vi "EE_DataAcquisitionLoop.vi"(8 "error in (no error)":errorcluster, 9 "StopButton Ref":refnum<vi>, 10 "RawDataQueue in":T1, 11 "EmotivEpocHeadsetControls in":refnum<class "EmotivEpocHeadsetControls.lvclass">) -> (0 "error out":errorcluster, 2 "RawDataQueue out":T1, 3 "EmotivEpocHeadsetControls out":refnum<class "EmotivEpocHeadsetControls.lvclass">)   [LabVIEW 2016, in "Emotiv Epoc.lvlib" / "EmotivEpocHeadsetControls.lvclass"]
uses:
  EmotivEpocHeadsetControls.lvclass
  EE_Queue_Refnum.ctl
  EE_Queue_Data_Type.ctl
  EE_SignalStrength_enum.ctl
  EE_EEG_ContactQuality_enum.ctl
  EmotivEpocHeadsetControls.lvclass/EmotivEpocHeadsetControls.ctl
  <vilib>/Platform/TimedLoop/XDataNode/timing_clust.ctl
  <vilib>/Platform/TimedLoop/XDataNode/nitl_modes.ctl
  <vilib>/Platform/TimedLoop/XDataNode/wakeup.ctl
  <vilib>/Platform/TimedLoop/XDataNode/XDataNode.xnode
  <vilib>/Platform/TimedLoop/XDataNode/XDNodeRunTimeDep.lvlib
  Emotiv Epoc.lvlib
panel:
  # "This VI is a part of BCI Design library, http://www.ru-bci.org \nCopyright © 2020, Sotnikov Peter, All rights reserved. License: CC BY-NC 4.0"
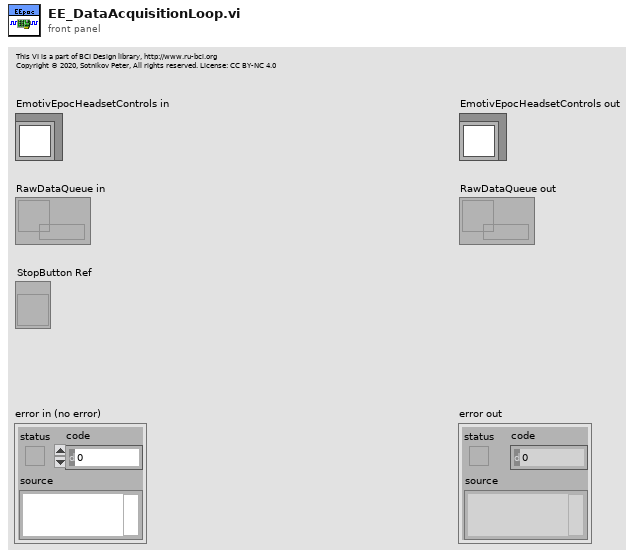
[diagram p1: front panel]
types:
  T1 = typedef "Emotiv Epoc.lvlib/EE_Queue_Refnum.ctl" = refnum<queue>
  T2 = typedef "Emotiv Epoc.lvlib/EE_Queue_Data_Type.ctl" = cluster{"FinishedLate?":bool, "UserActive?":bool, "WirelessSignalStatus":T3, "EDK_ERROR_CODE":i32, "nSampleOut":u32, "CurrentTimestamp":timestamp, "RawChannelsData ":dbl[][], "EEG_ContactsQuality":T4[]}
  T3 = typedef "Emotiv Epoc.lvlib/EmotivEpocHeadsetControls.lvclass/EE_SignalStrength_enum.ctl" = enum32{"NO_SIGNAL", "BAD_SIGNAL", "GOOD_SIGNAL"}
  T4 = typedef "Emotiv Epoc.lvlib/EE_EEG_ContactQuality_enum.ctl" = enum16{"EEG_CQ_NO_SIGNAL", "EEG_CQ_VERY_BAD", "EEG_CQ_POOR", "EEG_CQ_FAIR", "EEG_CQ_GOOD"}
  T5 = typedef "XDNodeRunTimeDep.lvlib/timing_clust.ctl" = cluster{"Expected End [f-1]":u64, "Actual End [f-1]":u64, "Finished Late? [f-1]":bool, "Expected End [i-1]":u64, "Actual End [i-1]":u64, "Finished Late? [i-1]":bool, "Expected Start [i]":u64, "Actual Start [i]":u64, "Expected Start [f]":u64, "Actual Start [f]":u64, "Source Name":string, "Structure Name":string, "Period":i64, "Deadline":i64, "Offset":i64, "Start":i64, "Priority":i32, "Timeout":i32, "Mode":T6, "Wakeup Reason":T7, "Error":errorcluster, "Source Type":string, "Secondary Source Type":string, "Global End Time":u64, "Global Start Time":u64, "Frame Duration":u64, "Iteration Duration":u64, "Assigned CPU":i32, "I/O Scan Engine Mode":u32}
  T6 = typedef "XDNodeRunTimeDep.lvlib/nitl_modes.ctl" = enum32{"No Change", "Process missed periods, maintain original phase", "Discard missed periods, maintain original phase", "Process missed periods, ignore original phase", "Discard missed periods, ignore original phase"}
  T7 = typedef "XDNodeRunTimeDep.lvlib/wakeup.ctl" = enum32{"Normal", "Aborted", "Asynchronous wakeup", "Timing source error", "Timed loop error", "Timeout"}
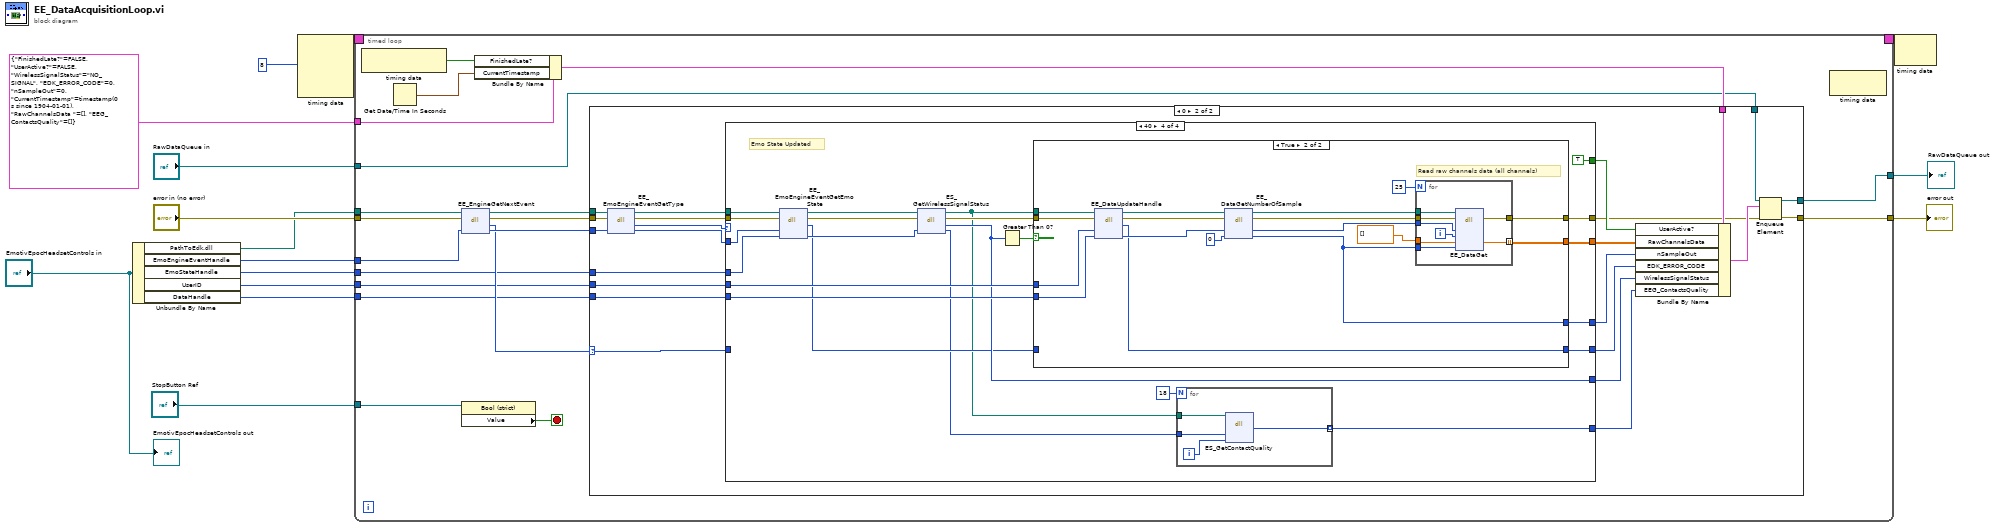
[diagram p0: block diagram]
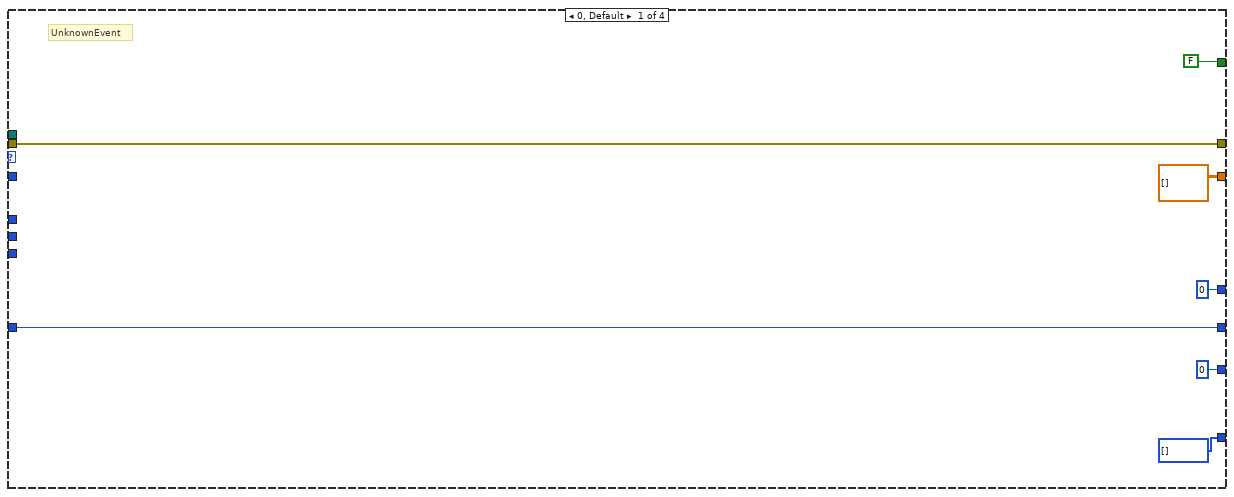
[diagram p3: hidden frame]
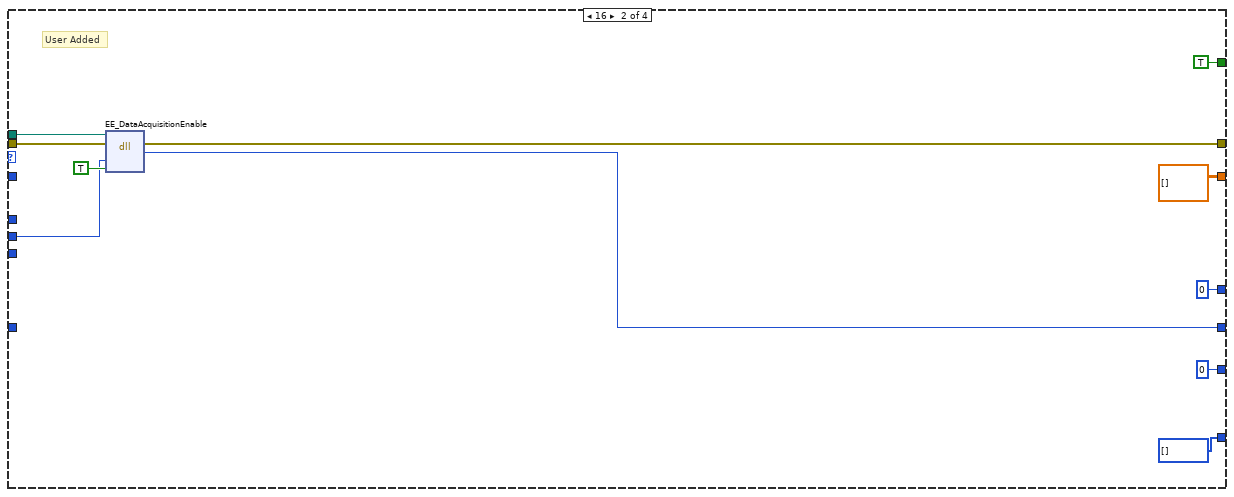
[diagram p4: hidden frame]
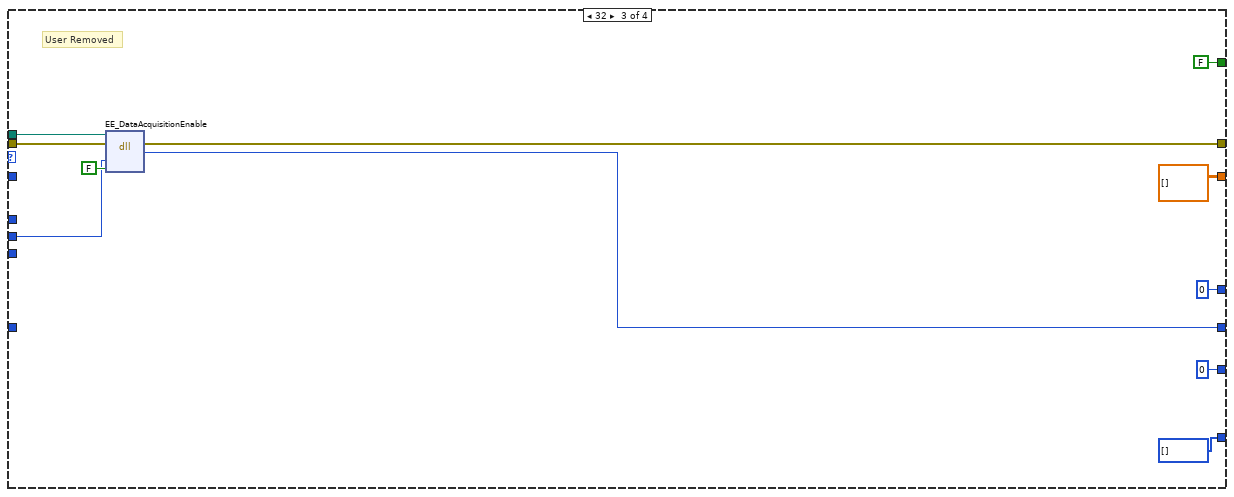
[diagram p5: hidden frame]
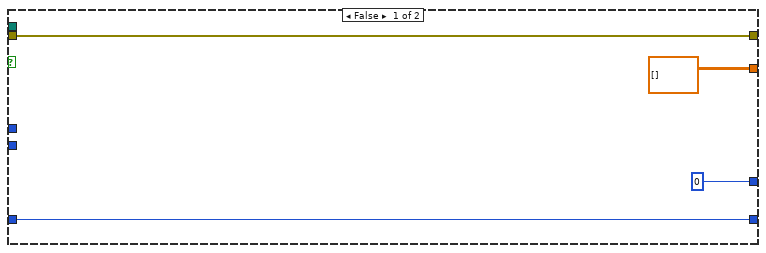
[diagram p6: hidden frame]
diagram:
  n1 = Unbundle By Name("EmotivEpocHeadsetControls in") -> ("PathToEdk.dll"=w10:path, "EmoEngineEventHandle"=w8:i64, "EmoStateHandle"=w5:i64, "UserID"=w6:u32, "DataHandle"=w4:i64)
  n2 = node-c288(i64 8 ("Period")) -> (w15:T5)  [unwired: 3 in]
  n3 = timed-loop {
    timing: w15 -> [_]
    timing-out: [_] -> w14
    tunnel: "error in (no error)" -> [w30]
    tunnel: "RawDataQueue in" -> [w18]
    tunnel: w10 -> [w29]
    tunnel: [w17] -> w9
    tunnel: w8 -> [w27]
    tunnel: "StopButton Ref" -> [w26]
    tunnel: w6 -> [w25]
    tunnel: w5 -> [w24]
    tunnel: w4 -> [w23]
    tunnel: T2 {"FinishedLate?"=FALSE, "UserActive?"=FALSE, "WirelessSignalStatus"=enum."NO_SIGNAL", "EDK_ERROR_CODE"=0, "nSampleOut"=0, "CurrentTimestamp"=timestamp(0 s since 1904-01-01), "RawChannelsData "=[], "EEG_ContactsQuality"=[]} ("Queue_Data_Type") -> [w22]
    tunnel: [w16] -> w1
    stop <- w34 stop-if-true
    n4 = node-c288() -> (w21:bool)  [unwired: 1 in]
    n5 = Get Date/Time In Seconds() -> (seconds since 1Jan1904=w20:timestamp)
    n6 = dll-call lib="?" fn="EE_EngineGetNextEvent"(path in=w29, error in=w30, "EmoEngineEventHandle"=w27) -> (path out=w32:path, error out=w31:errorcluster, "EDK_ERROR_CODE"=w28:i32, "EmoEngineEventHandle"=w33:i64)  [unwired: 1 in]
    n7 = property class="Bool (strict)"(reference=w26) -> ("Value"=w34:bool)  [unwired: 1 in, 2 out]
    n8 = Bundle By Name(cluster=w22, "FinishedLate?"=w21, "CurrentTimestamp"=w20) -> (w19:T2)
    n9 = case shown="0" w28 {
      selector: w28 -> [_ w49]
      tunnel: w33 -> [_ w55]
      tunnel: w32 -> [_ w54]
      tunnel: w31 -> [w36 w53]
      tunnel: [w36 w42] -> w17
      tunnel: w25 -> [_ w52]
      tunnel: w24 -> [_ w51]
      tunnel: w23 -> [_ w50]
      tunnel: w19 -> [_ w47]
      tunnel: w18 -> [w35 w46]
      tunnel: [w35 w45] -> w16
      frame 1536, Default {
        # "There are no new EmoEngine events at this time"
      }
      frame 0 {
        n10 = dll-call lib="C:/Program Files/Emotiv Development Kit_v1.0.0.3-PREMIUM/edk.dll" fn="EE_EmoEngineEventGetType"(path in=w54, error in=w53, "EmoEngineEventHandle"=w55) -> (path out=w58:path, error out=w57:errorcluster, "EE_Event_type"=w56:u32, "EmoEngineEventHandle"=w59:i64)  [unwired: 1 in]
        n11 = case shown="40" w56 {
          tunnel: w57 -> [w66 w77 w88 w110]
          tunnel: w58 -> [_ w76 w87 w109]
          tunnel: [w66 w75 w86 w102] -> w43
          tunnel: w59 -> [_ _ _ w104]
          tunnel: w52 -> [_ w73 w84 w99]
          tunnel: w51 -> [_ _ _ w101]
          tunnel: w50 -> [_ _ _ w100]
          tunnel: [u32 0 ("nSampleOut") u32 0 ("nSampleOut") u32 0 ("nSampleOut") w98] -> w41
          tunnel: [w63 w68 w80 w97] -> w39
          tunnel: [u32 0 ("EE_SignalStrength") u32 0 ("EE_SignalStrength") u32 0 ("EE_SignalStrength") w96] -> w38
          tunnel: [dbl[][] [] ("buffer") dbl[][] [] ("buffer") dbl[][] [] ("buffer") w94] -> w40
          tunnel: w49 -> [w63 _ _ _]
          tunnel: [FALSE TRUE FALSE TRUE] -> w44
          tunnel: [u8[] [] ("contactQuality") u8[] [] ("contactQuality") u8[] [] ("contactQuality") w89] -> w37
          frame 0, Default {
            # "UnknownEvent"
          }
          frame 16 {
            # "User Added"
            n12 = dll-call lib="?" fn="EE_DataAcquisitionEnable"(path in=w76, error in=w77, "userId"=w73, "enable"=TRUE ("Value")) -> (error out=w75:errorcluster, "EDK_ERROR_CODE"=w68:i32)  [unwired: 3 in, 1 out]
          }
          frame 32 {
            # "User Removed"
            n13 = dll-call lib="?" fn="EE_DataAcquisitionEnable"(path in=w87, error in=w88, "userId"=w84, "enable"=FALSE) -> (error out=w86:errorcluster, "EDK_ERROR_CODE"=w80:i32)  [unwired: 3 in, 1 out]
          }
          frame 64 {
            # "Emo State Updated"
            n14 = dll-call lib="C:/Program Files/Emotiv Development Kit_v1.0.0.3-PREMIUM/edk.dll" fn="EE_EmoEngineEventGetEmoState"(path in=w109, error in=w110, "EmoEngineEventHandle"=w104, "EmoStateHandle"=w101) -> (path out=w107:path, error out=w108:errorcluster, "EDK_ERROR_CODE"=w95:i32, "EmoStateHandle"=w106:i64)  [unwired: 2 in]
            n15 = dll-call lib="C:/Program Files/Emotiv Development Kit_v1.0.0.3-PREMIUM/edk.dll" fn="ES_GetWirelessSignalStatus"(path in=w107, error in=w108, "EmoStateHandle"=w106) -> (path out=w92:path, error out=w103:errorcluster, "EE_SignalStrength"=w96:i32, "EmoStateHandle"=w91:i64)  [unwired: 1 in]
            n16 = Greater Than 0?(x=w96) -> (x > 0?=w105:bool)
            n17 = case shown="True" w105 {
              tunnel: w103 -> [w118 w131]
              tunnel: [w118 w121] -> w102
              tunnel: w100 -> [_ w126]
              tunnel: w99 -> [_ w125]
              tunnel: [u32 0 ("nSampleOut") w123] -> w98
              tunnel: [w117 w122] -> w97
              tunnel: w95 -> [w117 _]
              tunnel: [dbl[][] [] ("buffer") w120] -> w94
              tunnel: w92 -> [_ w119]
              frame False {
              }
              frame True {
                # "Read raw channels data (all channels)"
                n18 = dll-call lib="?" fn="EE_DataUpdateHandle"(path in=w119, error in=w131, "userId"=w125, "hData"=w126) -> (path out=w133:path, error out=w132:errorcluster, "EDK_ERROR_CODE"=w122:i32, "hData"=w134:i64)  [unwired: 2 in]
                n19 = dll-call lib="?" fn="EE_DataGetNumberOfSample"(path in=w133, error in=w132, "hData"=w134, "nSampleOut"=u32 0) -> (path out=w128:path, error out=w127:errorcluster, "hData"=w130:i64, "nSampleOut"=w123:u32)  [unwired: 2 in]
                n20 = for {
                  N: 25 -> [_]
                  tunnel: w123 -> [w143]
                  tunnel: w130 -> [w142]
                  tunnel: [w141] -> w120 mode=indexing
                  tunnel: w128 -> [w140]
                  tunnel: w127 -> [w139]
                  tunnel: [w138] -> w121
                  tunnel: dbl[] [] -> [w136]
                  i -> [w137]
                  n21 = dll-call lib="?" fn="EE_DataGet"(path in=w140, error in=w139, "DataHandle"=w142, "EE_DataChannel_t"=w137, "buffer"=w136, "bufferSizeInSample"=w143) -> (error out=w138:errorcluster, "buffer"=w141:dbl[])  [unwired: 5 in, 1 out]
                }
              }
            }
            n22 = for {
              N: 18 -> [_]
              tunnel: w92 -> [w114]
              tunnel: w91 -> [w113]
              tunnel: [w111] -> w89 mode=indexing
              i -> [w112]
              n23 = dll-call lib="C:/Program Files (x86)/Emotiv Development Kit_v1.0.0.3-PREMIUM/edk.dll" fn="ES_GetContactQuality"(path in=w114, "EmoStateHandle"=w113, "electroIdx"=w112) -> ("EEG_ContactQuality"=w111:u16)  [unwired: 4 in, 2 out]
            }
          }
        }
        n24 = Bundle By Name(cluster=w47, "UserActive?"=w44, "RawChannelsData"=w40, "nSampleOut"=w41, "EDK_ERROR_CODE"=w39, "WirelessSignalStatus"=w38, "EEG_ContactsQuality"=w37) -> (w48:T2)
        n25 = Enqueue Element(queue=w46, element=w48, error in (no error)=w43) -> (queue out=w45:T1, error out=w42:errorcluster)  [unwired: 1 in, 1 out]
      }
    }
    n26 = node-c288() -> ()  [unwired: 1 in, 1 out]
  }
  "error out" <- w9
  "RawDataQueue out" <- w1
  n27 = node-c288(w14) -> ()  [unwired: 1 out]
  "EmotivEpocHeadsetControls out" <- "EmotivEpocHeadsetControls in"
